vi "SysDef.Search.Target.vi"(8 "error in (no error)":errorcluster, 11 "nodeID":u64) -> (0 "error out":errorcluster, 1 "Value out":u64, 3 "nodeID out":u64, 4 "Found?":bool)   [LabVIEW 2015, in "System Definition Utilities.lvlib"]
uses:
  System Definition Utilities.lvlib
  NationalInstruments.VeriStand.SystemDefinitionAPI
  <vilib>/NI Veristand/Custom Device Tools/Custom Device Utility Library/Custom Device Utility Library.lvlib
  NationalInstruments.VeriStand.SystemStorage
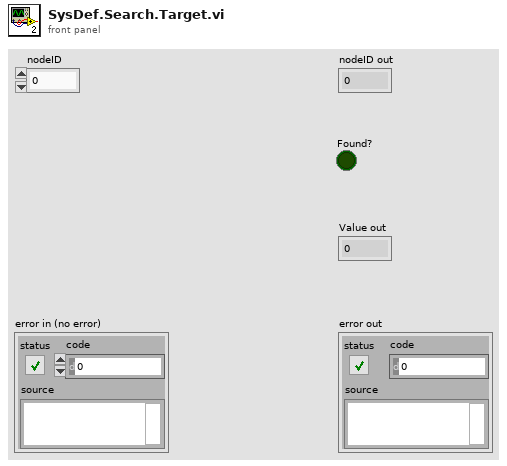
[diagram p1: front panel]
types:
  T1 = typedef "Custom Device API.lvlib/Custom Device Item Ref.ctl" = u64
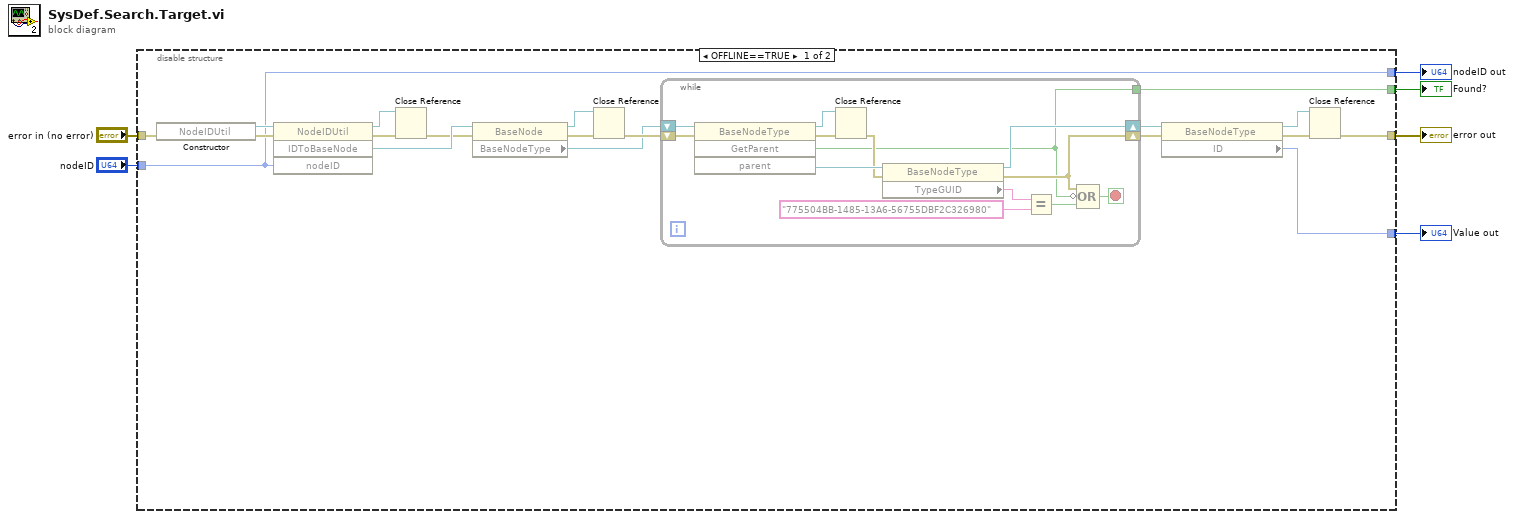
[diagram p0: block diagram]
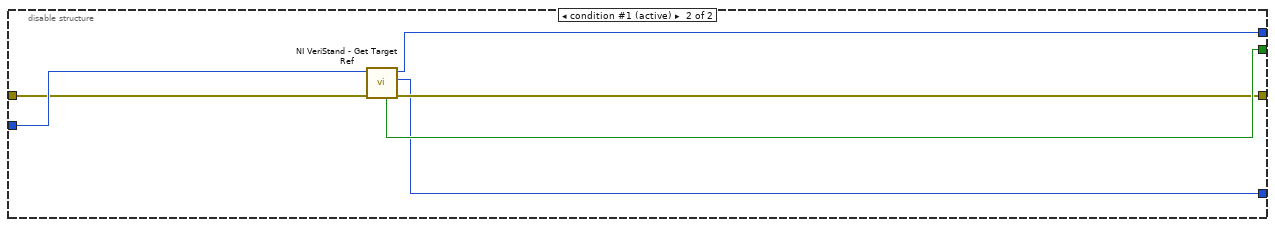
[diagram p2: hidden frame]
diagram:
  n1 = disable-structure shown="OFFLINE==TRUE" {
    disable-tunnel: "error in (no error)" -> [w19 w43]
    disable-tunnel: "nodeID" -> [w15 w44]
    disable-tunnel: [w16 w41] -> w4
    disable-tunnel: [w7 w42] -> w3
    disable-tunnel: [w8 w39] -> w2
    disable-tunnel: [w15 w40] -> w1
    frame condition #0 {
      n2 = constructor class="NodeIDUtil"(error in=w19) -> (reference out=w25:refnum<k24>, error out=w24:errorcluster)  [unwired: 2 in, 1 out]
      n3 = invoke class="NodeIDUtil" method="IDToBaseNode"(reference=w25, error in=w24, "nodeID"=w15) -> (reference out=w20:refnum<k24>, error out=w22:errorcluster, "IDToBaseNode"=w23:refnum<k24>)  [unwired: 1 in, 1 out]
      n4 = Close Reference(reference=w20, error in (no error)=w22) -> (error out=w21:errorcluster)
      n5 = property class="BaseNode"(reference=w23, error in=w21) -> (reference out=w18:refnum<k24>, error out=w17:errorcluster, "BaseNodeType"=w13:refnum<k24>)
      n6 = Close Reference(reference=w18, error in (no error)=w17) -> (error out=w14:errorcluster)
      n7 = while {
        shift-right: [w28] -> w10
        shift-left: w14 -> [w37]
        shift-right: [w27] -> w12
        shift-left: w13 -> [w38]
        tunnel: [w26] -> w7
        stop <- w34 stop-if-true
        n8 = invoke class="BaseNodeType" method="GetParent"(reference=w38, error in=w37) -> (reference out=w29:refnum<k24>, error out=w31:errorcluster, "GetParent"=w26:bool, "parent"=w36:refnum<k24>)  [unwired: 2 in]
        n9 = Close Reference(reference=w29, error in (no error)=w31) -> (error out=w30:errorcluster)
        n10 = property class="BaseNodeType"(reference=w36, error in=w30) -> (reference out=w27:refnum<k24>, error out=w28:errorcluster, "TypeGUID"=w32:string)
        n11 = Equal?(x=w32, y="775504BB-1485-13A6-56755DBF2C326980") -> (x = y?=w35:bool)
        n12 = Compound Arithmetic op=OR(w28, invert w26, w35) -> (w34:bool)
      }
      n13 = property class="BaseNodeType"(reference=w12, error in=w10) -> (reference out=w11:refnum<k24>, error out=w9:errorcluster, "ID"=w8:u64)
      n14 = Close Reference(reference=w11, error in (no error)=w9) -> (error out=w16:errorcluster)
    }
    frame condition #1 (active) {
      n15 = call <vilib>:"NI VeriStand - Get Target Ref.vi"("error in"=w43, "Item Ref in"=w44) -> ("error out"=w41:errorcluster, "Target Ref"=w39:T1, "Item Ref out"=w40:T1, "Found"=w42:bool)  [unwired: 6 in]
    }
  }
  "nodeID out" <- w1
  "error out" <- w4
  "Value out" <- w2
  "Found?" <- w3
